vi "sub vi - ReadPosition.vi"() -> (0 "Z Position":dbl, 1 "Y Position":dbl, 3 "X Position":dbl, 4 "X Voltage":dbl, 6 "Y Voltage":dbl, 8 "Z Voltage":dbl)   [LabVIEW 2010]
panel:
  # "About this Program:\n     - Reads the location of the Piezo location"
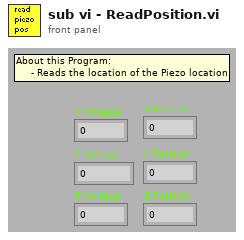
[diagram p1: front panel]
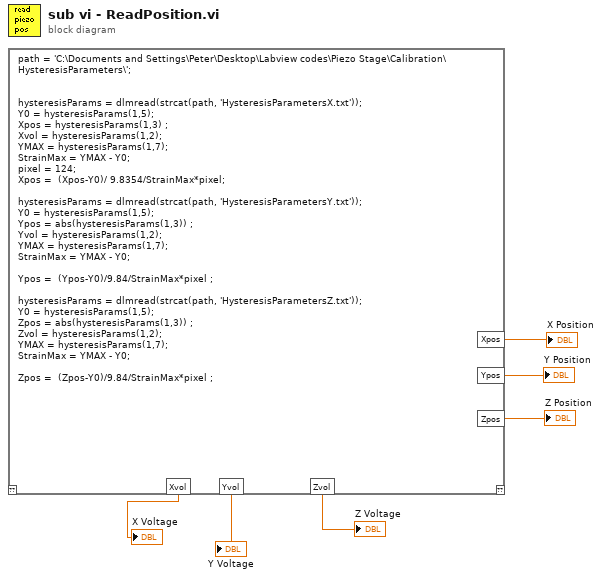
[diagram p0: block diagram]
diagram:
  n1 = script code="path = 'C:\\Documents and Settings\\Peter\\Desktop\\Labview codes\\Piezo Stage\\Calibration\\HysteresisParameters\\';\n\n\nhysteresisParams = dlmread(strcat(path, 'HysteresisParametersX.txt'));\nY0 = hysteresisParams(1,5);\nXpos = hysteresisParams(1,3) ;\nXvol = hysteresisParams(1,2);\nYMAX = hysteresisParams(1,7);\nStrainMax = YMAX - Y0;\npixel = 124;\nXpos =  (Xpos-Y0)/ 9.8354/StrainMax*pixel;\n\nhysteresisParams = dlmread(strcat(path, 'HysteresisParametersY.txt'));\nY0 = hysteresisParams(1,5);\nYpos = abs(hysteresisParams(1,3)) ;\nYvol = hysteresisParams(1,2);\nYMAX = hysteresisParams(1,7);\nStrainMax = YMAX - Y0;\n\nYpos =  (Ypos-Y0)/9.84/StrainMax*pixel ;\n\nhysteresisParams = dlmread(strcat(path, 'HysteresisParametersZ.txt'));\nY0 = hysteresisParams(1,5);\nZpos = abs(hysteresisParams(1,3)) ;\nZvol = hysteresisParams(1,2);\nYMAX = hysteresisParams(1,7);\nStrainMax = YMAX - Y0;\n\nZpos =  (Zpos-Y0)/9.84/StrainMax*pixel ;"() -> ("Xpos"=→"X Position":dbl, "Ypos"=→"Y Position":dbl, "Zpos"=→"Z Position":dbl, "Xvol"=→"X Voltage":dbl, "Yvol"=→"Y Voltage":dbl, "Zvol"=→"Z Voltage":dbl)  [unwired: 2 out]
